vi "Status TimerList (Core).vi"(7 "Timer Number":T5, 8 "error in (no error)":errorcluster, 10 "Address (0)":i32, 11 "VISA resource name":refnum<visa-resource-name>) -> (0 "error out":errorcluster, 1 "End Timer":T1 {"Start-Date (s)" format="%<%Y/%m/%d>T"; "Start-Time (s)" format="%<%H:%M>t"}, 2 "Start Timer":T1 {"Start-Date (s)" format="%<%Y/%m/%d>T"; "Start-Time (s)" format="%<%H:%M>t"}, 3 "VISA resource name out":refnum<visa-resource-name>, 5 "Quick Timer":T4 {"Set-Time (s)" format="%<%H:%M>t"})   [LabVIEW 2016, in "Environment Chamber.lvlib" / "Climatic Chamber.lvlib"]
doc: "<b>Timer content monitor</b>\n\nReturns the settings of the selected timer number. (Quick Timer, Start Timer, End Timer)"
uses:
  Climatic Chamber.lvlib
  Private/Type Defs/TimerNumber Enum.ctl
  Private/Type Defs/QuickTimer Cluster.ctl
  Private/Type Defs/Operation_Stop Mode Enum.ctl
  Private/Type Defs/Start_End Timer Cluster.ctl
  Private/Type Defs/Start Mode Enum.ctl
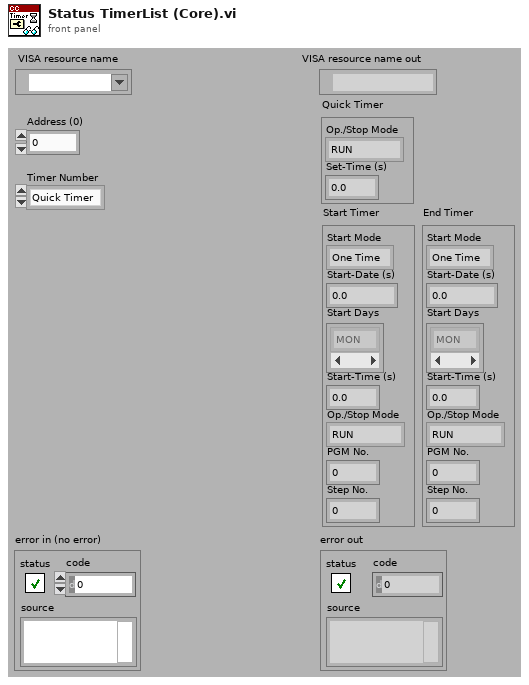
[diagram p1: front panel]
types:
  T1 = typedef "Environment Chamber.lvlib/Climatic Chamber.lvlib/Start_End Timer Cluster.ctl" = cluster{"Start Mode":T2, "Start-Date (s)":dbl, "Start Days":enum16{"MON", "TUE", "WED", "THU", "FRI", "SAT", "SUN"}[], "Start-Time (s)":dbl, "Op./Stop Mode":T3, "PGM No.":i32, "Step No.":i32}
  T2 = typedef "Environment Chamber.lvlib/Climatic Chamber.lvlib/Start Mode Enum.ctl" = enum16{"One Time", "Weekly", "Daily"}
  T3 = typedef "Environment Chamber.lvlib/Climatic Chamber.lvlib/Operation_Stop Mode Enum.ctl" = enum16{"RUN", "CONSTANT", "STANDBY", "OFF"}
  T4 = typedef "Environment Chamber.lvlib/Climatic Chamber.lvlib/QuickTimer Cluster.ctl" = cluster{"Op./Stop Mode":T3, "Set-Time (s)":dbl}
  T5 = typedef "Environment Chamber.lvlib/Climatic Chamber.lvlib/TimerNumber Enum.ctl" = enum16{"Quick Timer", "Start Timer", "End Timer"}
  T6 = enum16{"MON", "TUE", "WED", "THU", "FRI", "SAT", "SUN"}[]
  T7 = cluster{"Start Mode":T2, dbl, "Start Days":enum16{"MON", "TUE", "WED", "THU", "FRI", "SAT", "SUN"}[], dbl, "Op./Stop Mode Out":T3, "PGM No.":i32, "Step No.":i32}
  T8 = cluster{"Start Mode":T2, dbl, "Start/End Days":enum16{"MON", "TUE", "WED", "THU", "FRI", "SAT", "SUN"}[], dbl, "Op./Stop Mode Out":T3, "PGM No.":i32, "Step No.":i32}
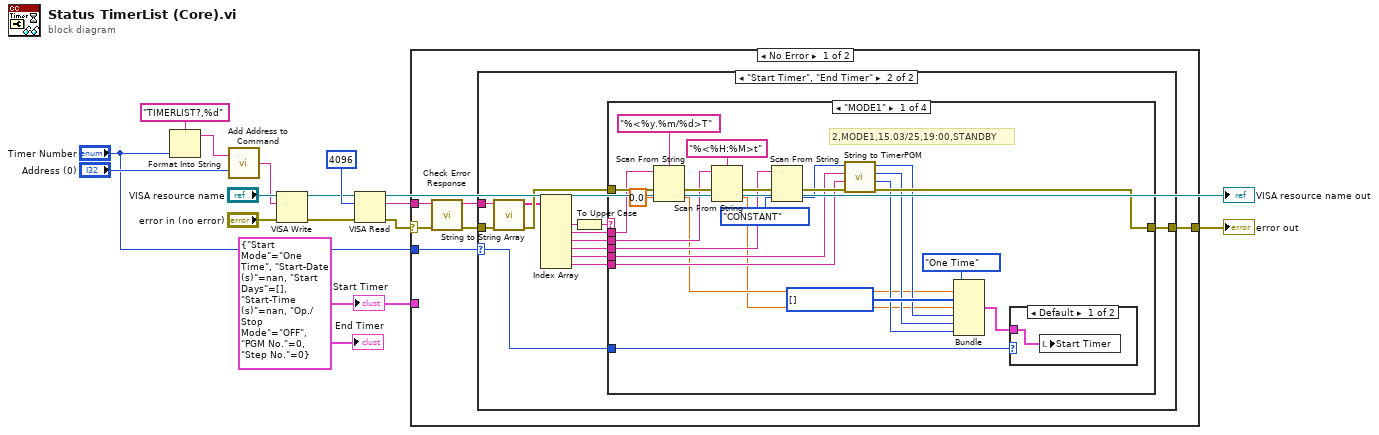
[diagram p0: block diagram]
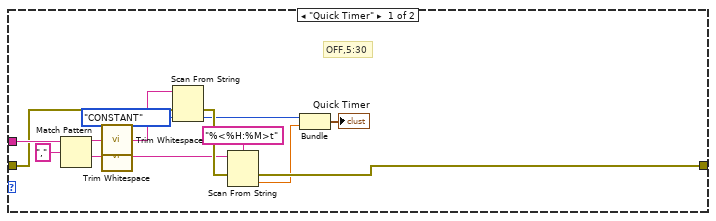
[diagram p2: hidden frame]
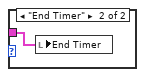
[diagram p3: hidden frame]
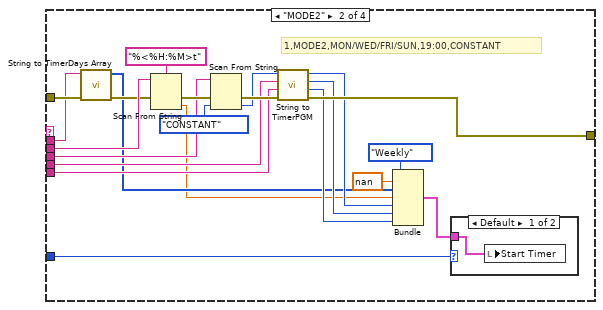
[diagram p4: hidden frame]
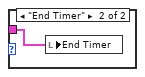
[diagram p5: hidden frame]
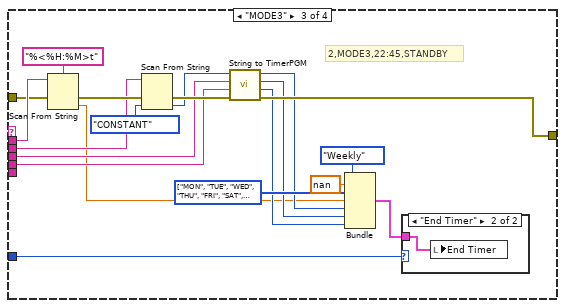
[diagram p6: hidden frame]
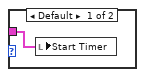
[diagram p7: hidden frame]
diagram:
  w1 = T1 {"Start Mode"=enum."One Time", "Start-Date (s)"=nan, "Start Days"=[], "Start-Time (s)"=nan, "Op./Stop Mode"=enum."OFF", "PGM No."=0, "Step No."=0} ("Start Timer")
  n1 = Format Into String(format string="TIMERLIST?,%d", "Timer Number") -> (resulting string=w3:string)  [unwired: 2 in, 1 out]
  n2 = call "Add Address to Command.vi"("Address (0)"="Address (0)", "Command"=w3) -> ("Command OUT"=w8:string)
  n3 = VISA Write(VISA resource name="VISA resource name", write buffer=w8, error in (no error)="error in (no error)") -> (VISA resource name out=w12:refnum<visa-resource-name>, error out=w11:errorcluster)  [unwired: 1 out]
  n4 = VISA Read(VISA resource name=w12, byte count=u32 4096, error in (no error)=w11) -> (VISA resource name out=→"VISA resource name out":refnum<visa-resource-name>, read buffer=w6:string, error out=w7:errorcluster)  [unwired: 1 out]
  n5 = case shown="No Error" w7 {
    selector: w7 -> [w20 w121]
    tunnel: w6 -> [w21 _]
    tunnel: [w16 w121] -> w5
    tunnel: "Timer Number" -> [w18 _]
    tunnel: w1 -> [_ _]
    frame No Error {
      n6 = call "Check Error Response.vi"("error in (no error)"=w20, "read String"=w21) -> ("error out"=w19:errorcluster, "String out"=w17:string)  [unwired: 7 in, 1 out]
      n7 = case shown="\"Start Timer\", \"End Timer\"" w18 {
        selector: w18 -> [_ w38]
        tunnel: w19 -> [w26 w46]
        tunnel: w17 -> [w33 w47]
        tunnel: [w35 w39] -> w16
        frame "Quick Timer" {
          # "OFF,5:30"
          n8 = Match Pattern(string=w33, regular expression=",") -> (before substring=w31:string, after substring=w30:string)  [unwired: 1 in, 2 out]
          n9 = call <vilib>:"Trim Whitespace.vi"("string"=w31) -> ("trimmed string"=w29:string)  [unwired: 1 in]
          n10 = call <vilib>:"Trim Whitespace.vi"("string"=w30) -> ("trimmed string"=w25:string)  [unwired: 1 in]
          n11 = Scan From String(input string=w29, error in=w26, default 1=Operation_Stop_Mode_Enum."CONSTANT" ("Op./Stop Mode")) -> (error out=w34:errorcluster, output 1=w27:T3)  [unwired: 2 in, 2 out]
          n12 = Scan From String(format string="%<%H:%M>t", input string=w25, error in=w34) -> (error out=w35:errorcluster, output 1=w23:dbl)  [unwired: 2 in, 2 out]
          n13 = Bundle("Op./Stop Mode"=w27, w23) -> (→"Quick Timer":cluster{"Op./Stop Mode":T3, dbl})  [unwired: 1 in]
        }
        frame "Start Timer", "End Timer" {
          n14 = call "String to String Array.vi"("error in (no error)"=w46, "String received"=w47) -> ("error out"=w48:errorcluster, "Array Data"=w45:string[])  [unwired: 8 in]
          n15 = Index Array(array=w45) -> (element #2=w44:string, element #3=w42:string, element #4=w41:string, element #5=w40:string, element #6=w37:string, element #7=w36:string)  [unwired: 7 in, 1 out]
          n16 = To Upper Case(1:w44) -> (0:w43:string)
          n17 = case shown="\"MODE1\"" w43 {
            tunnel: w42 -> [w69 w85 w110 _]
            tunnel: w41 -> [w65 w95 w108 _]
            tunnel: w40 -> [w64 w94 w101 _]
            tunnel: w48 -> [w72 w87 w109 _]
            tunnel: [w71 w83 w105 _] -> w39
            tunnel: w38 -> [w59 w89 w112 _]
            tunnel: w37 -> [w54 w78 w100 _]
            tunnel: w36 -> [w53 w77 _ _]
            frame "MODE1" {
              w58 = T6 [] items=["MON", "TUE", "WED", "THU", "FRI", "SAT", "SUN"] ("Start Days")
              # "2,MODE1,15.03/25,19:00,STANDBY"
              n18 = Scan From String(format string="%<%y.%m/%d>T", input string=w69, error in=w72, default 1=0.0) -> (error out=w66:errorcluster, output 1=w50:dbl)  [unwired: 1 in, 2 out]
              n19 = Scan From String(format string="%<%H:%M>t", input string=w65, error in=w66) -> (error out=w70:errorcluster, output 1=w49:dbl)  [unwired: 2 in, 2 out]
              n20 = Scan From String(input string=w64, error in=w70, default 1=Operation_Stop_Mode_Enum."CONSTANT" ("Op./Stop Mode")) -> (error out=w57:errorcluster, output 1=w56:T3)  [unwired: 2 in, 2 out]
              n21 = call "String to TimerPGM.vi"("error in"=w57, "Step String"=w53, "PGM String"=w54, "Op./Stop Mode"=w56) -> ("error out"=w71:errorcluster, "Step No."=w51:i32, "PGM No."=w52:i32, "Op./Stop Mode Out"=w55:T3)  [unwired: 4 in]
              n22 = Bundle("Start Mode"=Start_Mode_Enum."One Time", w50, "Start Days"=w58, w49, "Op./Stop Mode Out"=w55, "PGM No."=w52, "Step No."=w51) -> (w60:T7)  [unwired: 1 in]
              n23 = case shown="Default" w59 {
                tunnel: w60 -> [w73 w74]
                frame Default {
                  n24 = local write "Start Timer"(w73) -> ()
                }
                frame "End Timer" {
                  n25 = local write "End Timer"(w74) -> ()
                }
              }
            }
            frame "MODE2" {
              # "1,MODE2,MON/WED/FRI/SUN,19:00,CONSTANT"
              n26 = call "String to TimerDays Array.vi"("error in (no error)"=w87, "Timer Days"=w85) -> ("error out"=w86:errorcluster, "Start/End Days"=w76:T6)  [unwired: 8 in]
              n27 = Scan From String(format string="%<%H:%M>t", input string=w95, error in=w86) -> (error out=w96:errorcluster, output 1=w75:dbl)  [unwired: 2 in, 2 out]
              n28 = Scan From String(input string=w94, error in=w96, default 1=Operation_Stop_Mode_Enum."CONSTANT" ("Op./Stop Mode")) -> (error out=w84:errorcluster, output 1=w82:T3)  [unwired: 2 in, 2 out]
              n29 = call "String to TimerPGM.vi"("error in"=w84, "Step String"=w77, "PGM String"=w78, "Op./Stop Mode"=w82) -> ("error out"=w83:errorcluster, "Step No."=w79:i32, "PGM No."=w80:i32, "Op./Stop Mode Out"=w81:T3)  [unwired: 4 in]
              n30 = Bundle("Start Mode"=Start_Mode_Enum."Weekly", nan, "Start/End Days"=w76, w75, "Op./Stop Mode Out"=w81, "PGM No."=w80, "Step No."=w79) -> (w90:T8)  [unwired: 1 in]
              n31 = case shown="Default" w89 {
                tunnel: w90 -> [w97 w98]
                frame Default {
                  n32 = local write "Start Timer"(w97) -> ()
                }
                frame "End Timer" {
                  n33 = local write "End Timer"(w98) -> ()
                }
              }
            }
            frame "MODE3" {
              w107 = T6 [enum."MON", enum."TUE", enum."WED", enum."THU", enum."FRI", enum."SAT", enum."SUN"] items=["MON", "TUE", "WED", "THU", "FRI", "SAT", "SUN"] ("Start/End Days")
              # "2,MODE3,22:45,STANDBY"
              n34 = Scan From String(format string="%<%H:%M>t", input string=w110, error in=w109) -> (error out=w117:errorcluster, output 1=w99:dbl)  [unwired: 2 in, 2 out]
              n35 = Scan From String(input string=w108, error in=w117, default 1=Operation_Stop_Mode_Enum."CONSTANT" ("Op./Stop Mode")) -> (error out=w118:errorcluster, output 1=w106:T3)  [unwired: 2 in, 2 out]
              n36 = call "String to TimerPGM.vi"("error in"=w118, "Step String"=w100, "PGM String"=w101, "Op./Stop Mode"=w106) -> ("error out"=w105:errorcluster, "Step No."=w102:i32, "PGM No."=w103:i32, "Op./Stop Mode Out"=w104:T3)  [unwired: 4 in]
              n37 = Bundle("Start Mode"=Start_Mode_Enum."Weekly", nan, "Start/End Days"=w107, w99, "Op./Stop Mode Out"=w104, "PGM No."=w103, "Step No."=w102) -> (w113:T8)  [unwired: 1 in]
              n38 = case shown="\"End Timer\"" w112 {
                tunnel: w113 -> [w119 w120]
                frame Default {
                  n39 = local write "Start Timer"(w119) -> ()
                }
                frame "End Timer" {
                  n40 = local write "End Timer"(w120) -> ()
                }
              }
            }
            frame Default {
            }
          }
        }
      }
    }
    frame Error {
    }
  }
  "error out" <- w5
  "Start Timer" <- w1
  "End Timer" <- w1
